vi "Receive Message.vi"(6 "priority":i32, 10 "IModel in":refnum<class "IModel.lvclass">, 11 "Message in":refnum<class "Message.lvclass">) -> (0 "error out":errorcluster, 2 "Actor out":refnum<class "Actor.lvclass">)   [LabVIEW 2018, in "MVA Framework.lvlib" / "IModel.lvlib" / "IModel.lvclass"]
doc: "This VI should be overriden ONLY if you are creating a proxy actor for remote transmission. If you are, override this VI to transmit the received message to a new destination, maintaining the given priority."
uses:
  IModel.lvclass
  <vilib>/ActorFramework/Stop Msg/Stop Msg.lvclass
  IObserver/IObserver/IObserver.lvclass
  C:/Program Files (x86)/National Instruments/LabVIEW 2020/vi.lib/ActorFramework/Message/Message.lvclass
  C:/Program Files (x86)/National Instruments/LabVIEW 2020/vi.lib/ActorFramework/Actor/Actor.lvclass
  <vilib>/ActorFramework/Actor/Actor.lvclass
  <vilib>/ActorFramework/Message/Message.lvclass
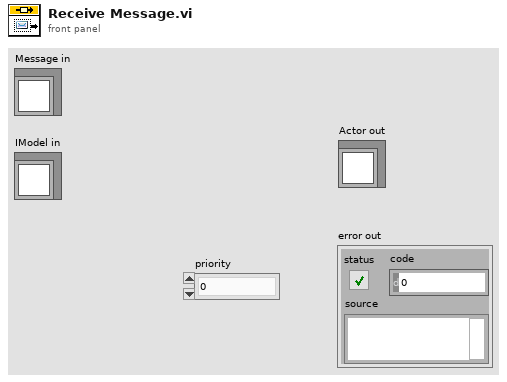
[diagram p1: front panel]
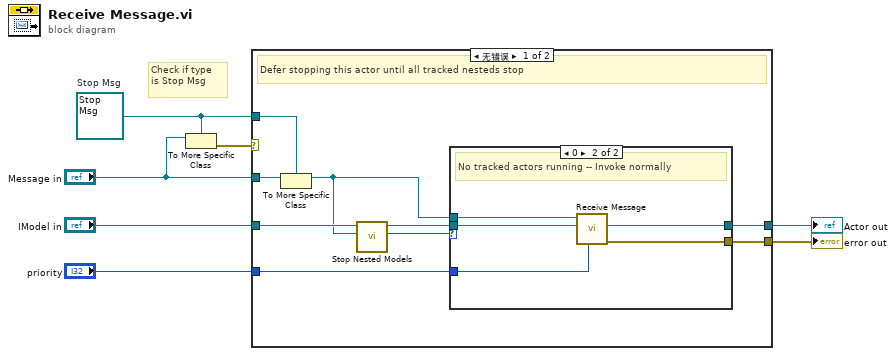
[diagram p0: block diagram]
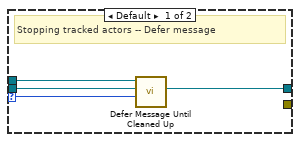
[diagram p2: hidden frame]
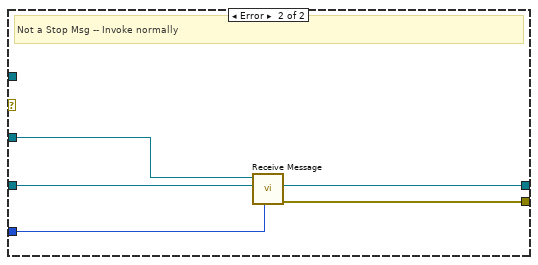
[diagram p3: hidden frame]
diagram:
  w1 = refnum<class "Stop Msg.lvclass"> refnum  # Stop Msg
  # "Check if type\nis Stop Msg"
  n1 = To More Specific Class(target class=w1, reference="Message in") -> (error out=w3:errorcluster)  [unwired: 1 in, 1 out]
  n2 = case shown="无错误" w3 {
    tunnel: [w16 w30] -> w7
    tunnel: [w14 w29] -> w6
    tunnel: "priority" -> [w12 w28]
    tunnel: "IModel in" -> [w15 w27]
    tunnel: "Message in" -> [w13 w26]
    tunnel: w1 -> [w9 _]
    frame No Error {
      # "Defer stopping this actor until all tracked nesteds stop"
      n3 = To More Specific Class(target class=w9, reference=w13) -> (specific class reference=w8:refnum<class "Stop Msg.lvclass">)  [unwired: 1 in, 1 out]
      n4 = call "Stop Nested Models.vi"("Stop Msg"=w8, "IModel in"=w15) -> ("Tracked Actors Running"=w10:i32, "IModel out"=w11:refnum<class "IModel.lvclass">)  [unwired: 7 in, 1 out]
      n5 = case shown="0" w10 {
        selector: w10 -> [w17 _]
        tunnel: [_ w23] -> w16
        tunnel: [w20 w24] -> w14
        tunnel: w8 -> [w19 w25]
        tunnel: w12 -> [_ w22]
        tunnel: w11 -> [w18 w21]
        frame Default {
          # "Stopping tracked actors -- Defer message"
          n6 = call "Defer Message Until Cleaned Up.vi"("Tracked Actor Count"=w17, "IModel in"=w18, "Message in"=w19) -> ("IModel out"=w20:refnum<class "IModel.lvclass">)  [unwired: 8 in]
        }
        frame 0 {
          # "No tracked actors running -- Invoke normally"
          n7 = call-parent "Receive Message.vi"("priority"=w22, "Actor in"=w21, "Message in"=w25) -> ("error out"=w23:errorcluster, "Actor out"=w24:refnum<class "Actor.lvclass">)  [unwired: 7 in]
        }
      }
    }
    frame Error {
      # "Not a Stop Msg -- Invoke normally"
      n8 = call-parent "Receive Message.vi"("priority"=w28, "Actor in"=w27, "Message in"=w26) -> ("error out"=w30:errorcluster, "Actor out"=w29:refnum<class "Actor.lvclass">)  [unwired: 7 in]
    }
  }
  "error out" <- w7
  "Actor out" <- w6
